vi "IQ Impairments impl.vi"(0 "session in":T1 {"rx baseband session"."3630 session"."Address Space" items=["VXI/VME A16"=1, "VXI/VME A24"=2, "VXI/VME A32"=3, "VXI/VME A64"=4, "PXI Memory Allocations"=9, "PXI Configuration"=10, "PXI BAR0"=11, "PXI BAR1"=12, "PXI BAR2"=13, "PXI BAR3"=14, "PXI BAR4"=15, "PXI BAR5"=16]; "tx baseband session"."3610 session"."Address Space" items=["VXI/VME A16"=1, "VXI/VME A24"=2, "VXI/VME A32"=3, "VXI/VME A64"=4, "PXI Memory Allocations"=9, "PXI Configuration"=10, "PXI BAR0"=11, "PXI BAR1"=12, "PXI BAR2"=13, "PXI BAR3"=14, "PXI BAR4"=15, "PXI BAR5"=16]}, 1 "direction":T12, 7 "device configuration":T15 {"Tx hardware configuration"."frequency (Hz)" format="%#_6p"; "Rx hardware configuration"."frequency (Hz)" format="%#_6p"}, 9 "IQ Impairments":T18[](array[typedef]) {"Phase Offset (radians)" format="%#_6f"; "Gain Imbalance (linear)" format="%#_6f"}, 11 "error in (no error)":errorcluster) -> (3 "scope":string[](array[string]), 4 "session out":T1 {"rx baseband session"."3630 session"."Address Space" items=["VXI/VME A16"=1, "VXI/VME A24"=2, "VXI/VME A32"=3, "VXI/VME A64"=4, "PXI Memory Allocations"=9, "PXI Configuration"=10, "PXI BAR0"=11, "PXI BAR1"=12, "PXI BAR2"=13, "PXI BAR3"=14, "PXI BAR4"=15, "PXI BAR5"=16]; "tx baseband session"."3610 session"."Address Space" items=["VXI/VME A16"=1, "VXI/VME A24"=2, "VXI/VME A32"=3, "VXI/VME A64"=4, "PXI Memory Allocations"=9, "PXI Configuration"=10, "PXI BAR0"=11, "PXI BAR1"=12, "PXI BAR2"=13, "PXI BAR3"=14, "PXI BAR4"=15, "PXI BAR5"=16]}, 6 "configuration gain":dbl[](array[numeric]), 8 "Index":i32[](array[numeric]), 14 "gain (db)":dbl[](array[numeric]), 15 "error out":errorcluster)   [LabVIEW 2019]
uses:
  <instrlib>/niMmWave/ni3620/Config/v1/Host/Public/Corrections/Typedefs/Opera IQ Impairment Data.ctl
  TypeDefs/Direction.ctl
  TypeDefs/Front End Configuration.ctl
  TypeDefs/Channel Configuration.ctl
  <instrlib>/niMmWave/ni3620/Config/v1/Host/Public/Typedefs/mmWave Port.ctl
  TypeDefs/Session.ctl
  <instrlib>/niMmWave/ni3620/Config/v1/Host/Public/High-Level/niMmWave Session.ctl
  <instrlib>/_niInstr/Register Bus/v0/Host/Public/Register Bus Session.ctl
  <instrlib>/_niInstr/Register Bus/v0/Host/Private/Session Data.ctl
  <instrlib>/niMmWave/ni3620/Config/v1/Host/Public/Typedefs/Board Information.ctl
  <instrlib>/niMmWave/ni3620/Config/v1/Host/Public/Typedefs/Hardware Revision.ctl
  <instrlib>/niMmWave/ni3620/Config/v1/Host/Public/Typedefs/Gain Mapping.ctl
  <instrlib>/niMmWave/ni3620/Config/v1/Host/Public/Typedefs/Correction Data.ctl
  <instrlib>/niMmWave/ni3620/Config/v1/Host/Public/Typedefs/Opera Characterization.ctl
  <instrlib>/niMmWave/ni3620/Config/v1/Host/Public/Corrections/Typedefs/Opera Characterization Main Header.ctl
  <instrlib>/niMmWave/ni3620/Config/v1/Host/Public/Corrections/Typedefs/Opera IF Board Information.ctl
  <instrlib>/niMmWave/ni3620/Config/v1/Host/Public/Corrections/Typedefs/Opera Characterization Instance Header.ctl
  <instrlib>/niMmWave/ni3620/Config/v1/Host/Public/Corrections/Typedefs/Opera Characterization Device Data Header.ctl
  <instrlib>/niMmWave/ni3620/Config/v1/Host/Public/Corrections/Typedefs/Opera LO Characterization Data Header.ctl
  <instrlib>/niMmWave/ni3620/Config/v1/Host/Public/Corrections/Typedefs/Opera IF Board Characterization Data Header.ctl
  <instrlib>/niMmWave/ni3620/Config/v1/Host/Public/Corrections/Typedefs/Opera Characterization Device Data.ctl
  <instrlib>/niMmWave/ni3620/Config/v1/Host/Public/Corrections/Typedefs/Opera LO2 Board Characterization Data.ctl
  <instrlib>/niMmWave/ni3620/Config/v1/Host/Public/Corrections/Typedefs/Opera LO Characterization Data.ctl
  <instrlib>/niMmWave/ni3620/Config/v1/Host/Public/Corrections/Typedefs/Opera IF Board Characterization Data.ctl
  <instrlib>/niMmWave/ni3620/Config/v1/Host/Public/Typedefs/mmWave Adapter Session Data.ctl
  <instrlib>/niMmWave/ni3620/Config/v1/Host/Public/Typedefs/mmWave Adapter Data.ctl
  <instrlib>/niMmWave/ni3620/Config/v1/Host/Public/Typedefs/mmWave Adapter 2.ctl
  <instrlib>/niMmWave/ni3620/Config/v1/Shared/Typedefs/Subsystem ID.ctl
  <instrlib>/niMmWave/ni3620/Config/v1/Host/Public/Typedefs/mmWave Adapter Channel Information.ctl
  <instrlib>/niMmWave/ni3620/Config/v1/Host/Public/Typedefs/Temperature Coefficients.ctl
  <instrlib>/niMmWave/ni3620/Config/v1/Host/Public/Typedefs/mmWave Characterization.ctl
  <instrlib>/niMmWave/ni3620/Config/v1/Host/Public/Corrections/Typedefs/mmWave Characterization Main Header.ctl
  <instrlib>/niMmWave/ni3620/Config/v1/Host/Public/Corrections/Typedefs/mmWave Characterization Instance Header.ctl
  <instrlib>/niMmWave/ni3620/Config/v1/Host/Public/Typedefs/Session Cache.ctl
  <instrlib>/niMmWave/ni3620/Config/v1/Host/Public/Typedefs/LO2 settings cache.ctl
  <instrlib>/niMmWave/ni3620/Config/v1/Host/Public/Typedefs/LO2 source.ctl
  <instrlib>/niMmWave/ni3620/Config/v1/Host/Public/Typedefs/Desired and Coerced.ctl
  <instrlib>/niMmWave/ni3620/Config/v1/Host/Public/Typedefs/Export cache.ctl
  <instrlib>/niMmWave/ni3620/Config/v1/Host/Public/Typedefs/Path cache.ctl
  <instrlib>/niMmWave/ni3620/Config/v1/Host/Public/Typedefs/Daughterboard Type.ctl
  <instrlib>/niMmWave/ni3620/Config/v1/Host/Public/Typedefs/LO1 settings cache.ctl
  <instrlib>/niMmWave/ni3620/Config/v1/Host/Public/Typedefs/LO1 Source.ctl
  <instrlib>/niMmWave/ni3620/Config/v1/Host/Public/Typedefs/mmWave export cache.ctl
  <instrlib>/niMmWave/ni3620/Config/v1/Host/Private/Board/LO2/LO2 Board Configuration Cache.ctl
  <instrlib>/niMmWave/ni3620/Config/v1/Host/Public/Typedefs/reference clock routing settings.ctl
  <instrlib>/niMmWave/ni3620/Config/v1/Host/Public/Typedefs/LO2 routing settings.ctl
  <instrlib>/niMmWave/ni3620/Config/v1/Host/Private/Board/LO1/LO1 Board Configuration Cache.ctl
  <instrlib>/niMmWave/ni3620/Config/v1/Host/Public/Typedefs/LO1 source settings.ctl
  <instrlib>/niMmWave/ni3620/Config/v1/Host/Public/Typedefs/LO1 export settings.ctl
  <instrlib>/niMmWave/ni3620/Config/v1/Host/Public/Typedefs/LO1 mmWave settings.ctl
  TypeDefs/Tx Baseband Session.ctl
  <instrlib>/niMmWave/ni3610 and ni3630/controls/public/Main Settings.ctl
  <vilib>/Instr/_visa.llb/VISA Register Access Address Space.ctl
  <instrlib>/niMmWave/ni3610 and ni3630/controls/public/Register Adresses.ctl
  <instrlib>/niMmWave/ni3610 and ni3630/controls/public/Base Card Type.ctl
  <instrlib>/niMmWave/ni3610 and ni3630/controls/private/IQ Card Revision.ctl
  <instrlib>/niMmWave/ni3610 and ni3630/controls/public/Board Capability.ctl
  TypeDefs/Blank FPGA Reference.ctl
  TypeDefs/Rx Baseband Session.ctl
  TypeDefs/Hardware Configuration.ctl
  TypeDefs/Gain Ranging.ctl
  TypeDefs/PXI Trigger Bus Info.ctl
  TypeDefs/Shared FPGA Reference.ctl
  <vilib>/Utility/error.llb/Error Cluster From Error Code.vi
  <vilib>/rvi/errors/niLvFpgaAdjustHostInterfaceError.vi
  <vilib>/rvi/interface/nirviReadWriteControl/nirviReadWriteControl.xnode
  NiFpgaLv.dll
  <vilib>/rvi/interface/Simulation/niFpgaSimulationCallBeginRW.vi
  <instrlib>/niMmWave/ni3620/Config/v1/Host/niMmWave Config v1 Host.lvlib
  <instrlib>/niMmWave/ni3620/Config/v1/Shared/niMmWave Config v1 Shared.lvlib
  <instrlib>/_niInstr/Register Bus/v0/Host/niInstr Register Bus v0 Host.lvlib
  <instrlib>/niMmWave/ni3610 and ni3630/ni3610_and_ni3630_Driver_Lib.lvlib
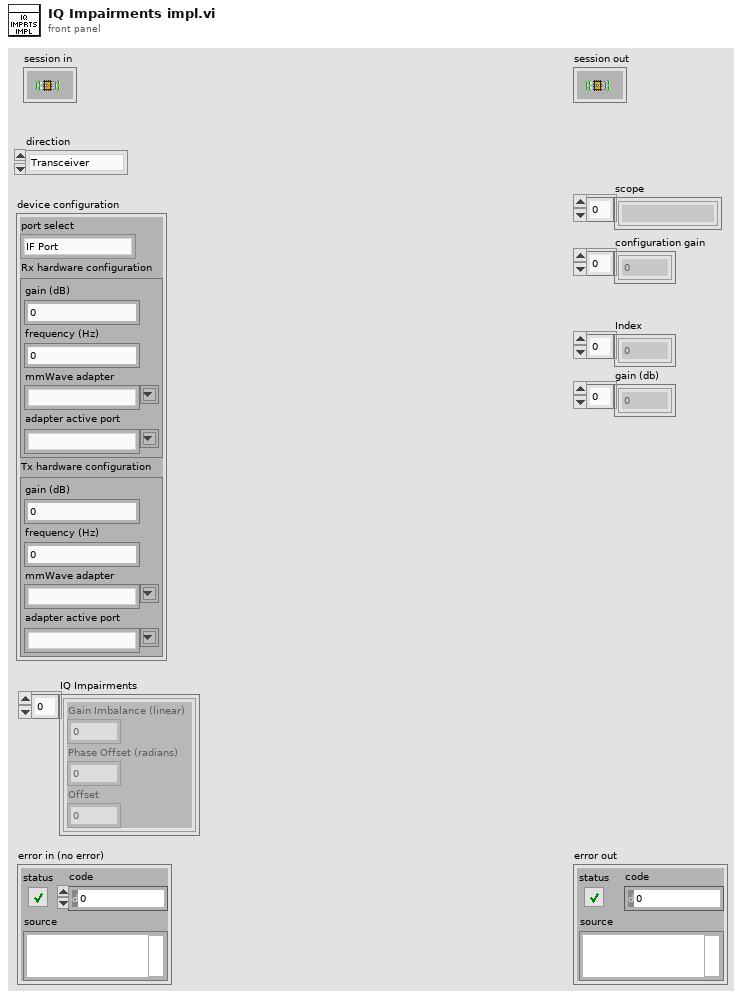
[diagram p1: front panel]
types:
  T1 = typedef "Session.ctl" = cluster{"3620 session":refnum<queue>, "tx baseband session":T2, "rx baseband session":T10, "tx gain (dB)":dbl, "rx gain (dB)":dbl, "hardware configuration":T11, "gain ranging":T13[], "pxi trigger bus information":T14}
  T2 = typedef "Tx Baseband Session.ctl" = cluster{"3610 session":T3, "7902 reference":T9}
  T3 = typedef "ni3610_and_ni3630_Driver_Lib.lvlib/Main Settings.ctl" = cluster{"VISA resource name":refnum<visa-resource-name>, "Address Space":T4, "window_offset":u32, "register_addresses":T5, "required_MM_fpga_version":cluster{"signature":u32, "hardware":u32, "current revision":u32, "oldest revision":u32}, "CPLD Oldest Compat Version ":cluster{"hardware":u32, "CPLD firmware":u32}, "MM_FPGA_image_location":string, "is_init":bool, "card_type":T6, "DacLmkConfigFileName":string, "AdcLmkConfigFileName":string, "AdcConfigFileName":string, "DacConfigFileName_RevA":string, "DacConfigFileName_RevB":string, "Mulde hardware revision":u8, "bypass DAC PLL\n":bool, "IQ Card Revision":T7, "board capability":T8}
  T4 = typedef "VISA Register Access Address Space.ctl" = u16
  T5 = typedef "ni3610_and_ni3630_Driver_Lib.lvlib/Register Adresses.ctl" = cluster{"MM based Registers":cluster{"Revision":u32, "OldestCompatRev":u32, "signature":u32, "scratch":u32, "LedControl":u32, "BoardHwRev":u32, "BoardControl":u32, "ThermalStatus":u32, "BasebandStatus":u32, "BasebandControl":u32, "BasebandAuxSetup":u32, "BasebandAuxStatus":u32, "LmkSyncOutSetup":u32, " AdcSyncOutSetup":u32, " InjSyncOutSetup":u32, " PxiTrig0OutSetup":u32, " PxiTrig1OutSetup":u32, " PxiTrig2OutSetup":u32, " PxiTrig3OutSetup":u32, " PxiTrig4OutSetup":u32, " PxiTrig5OutSetup":u32, " PxiTrig6OutSetup":u32, " PxiTrig7OutSetup":u32}, "CPLD based Registers":cluster{"SlaveSignature":u32, "SlaveRevision":u32, "SlaveOldestCompatRev":u32, "SlaveScratch":u32, "SlaveSetup":u32, "SlaveStatus":u32, "IDacReg_offset":u32, "LMKRegGrp0_offset":u32, "QDacReg_offset":u32, "BrdTempSensorVal":u32, "TempSensorPowerDown":u32, "GPIOReg_offset":u32, "IAdcReg_offset":u32, "QAdcReg_offset":u32, "LMKRegGrp1_offset":u32, "QadcTempSensorVal":u32, "IadcTempSensorVal":u32, "RevisionReg":u32, "VcxoReg":u32, "CpldStatusReg":u32, "PowerReg":u32, "VBiasEnReg":u32, "ExtRefOeReg":u32, "QdacCtrlReg":u32, "QdacStatusReg":u32, "IdacCtrlReg":u32, "IdacStatusReg":u32, "QdacJtagIn":u32, "QdacJtagOut":u32, "IdacJtagIn":u32, "IdacJtagOut":u32, "IqDcSetupReg":u32, "QadcStatusReg":u32, "IadcStatusReg":u32, "BrdSetupReg":u32, "IqDcRevisionReg":u32, "PllStatusReg":u32, "EndpointScratchReg":u32, "AdcSyncCfgReg":u32, "IqCardOpampReg":u32}, "CPLD Register Offset":u32, "MM  Register Offset":u32, " PxiTrig0OutSetup":u32}
  T6 = typedef "ni3610_and_ni3630_Driver_Lib.lvlib/Base Card Type.ctl" = enum16{"unspecified", "ADC", "DAC"}
  T7 = typedef "ni3610_and_ni3630_Driver_Lib.lvlib/IQ Card Revision.ctl" = enum16{"RevA", "RevB", "RevC", "RevD"}
  T8 = typedef "ni3610_and_ni3630_Driver_Lib.lvlib/Board Capability.ctl" = cluster{"baseband sync":enum16{"no baseband sync", "baseband sync"}}
  T9 = typedef "Blank FPGA Reference.ctl" = refnum<k20>
  T10 = typedef "Rx Baseband Session.ctl" = cluster{"3630 session":T3, "7902 reference":T9}
  T11 = typedef "Hardware Configuration.ctl" = cluster{"direction":T12, "baseband only":bool}
  T12 = typedef "Direction.ctl" = enum16{"Transceiver", "Receiver", "Transmitter"}
  T13 = typedef "Gain Ranging.ctl" = cluster{"gain ranging active scope":string, "gain ranging stream session":refnum<k20>}
  T14 = typedef "PXI Trigger Bus Info.ctl" = cluster{"chassis resource name":refnum<visa-resource-name>, "7902R (TX)":i16, "3610 (TX)":i16, "3620 (IF)":i16, "3630 (RX)":i16, "7902R (RX)":i16}
  T15 = typedef "Front End Configuration.ctl" = cluster{"port select":enum16{"IF Port", "Loopback", "Sync Port"}, "Rx hardware configuration":T16, "Tx hardware configuration":T16}
  T16 = typedef "Channel Configuration.ctl" = cluster{"gain (dB)":dbl, "frequency (Hz)":dbl, "mmWave adapter":string, "adapter active port":T17}
  T17 = typedef "niMmWave Config v1 Host.lvlib/mmWave Port.ctl" = string
  T18 = typedef "niMmWave Config v1 Host.lvlib/Opera IQ Impairment Data.ctl" = cluster{"Gain Imbalance (linear)":dbl, "Phase Offset (radians)":dbl, "Offset ":cdb}
  T19 = typedef "Shared FPGA Reference.ctl" = refnum<k20>
  T20 = cluster{"sample delay":cluster{"I delay":fxp<+,13,13>, "Q delay":fxp<+,13,13>}, "fractional delay":cluster{"enable":bool, "coef write":bool, "coef data":fxp<+/-,18,1>}, "impairments":cluster{"inline gain I":fxp<+/-,18,1>, "inline gain Q":fxp<+/-,18,1>, "cross gain I":fxp<+/-,18,1>, "cross gain Q":fxp<+/-,18,1>, "pre-gain offset I":fxp<+/-,18,1>, "pre-gain offset Q":fxp<+/-,18,1>, "post-gain offset I":fxp<+/-,18,1>, "post-gain offset Q":fxp<+/-,18,1>}, "iq inversion":cluster{"invert I":bool, "invert Q":bool}}
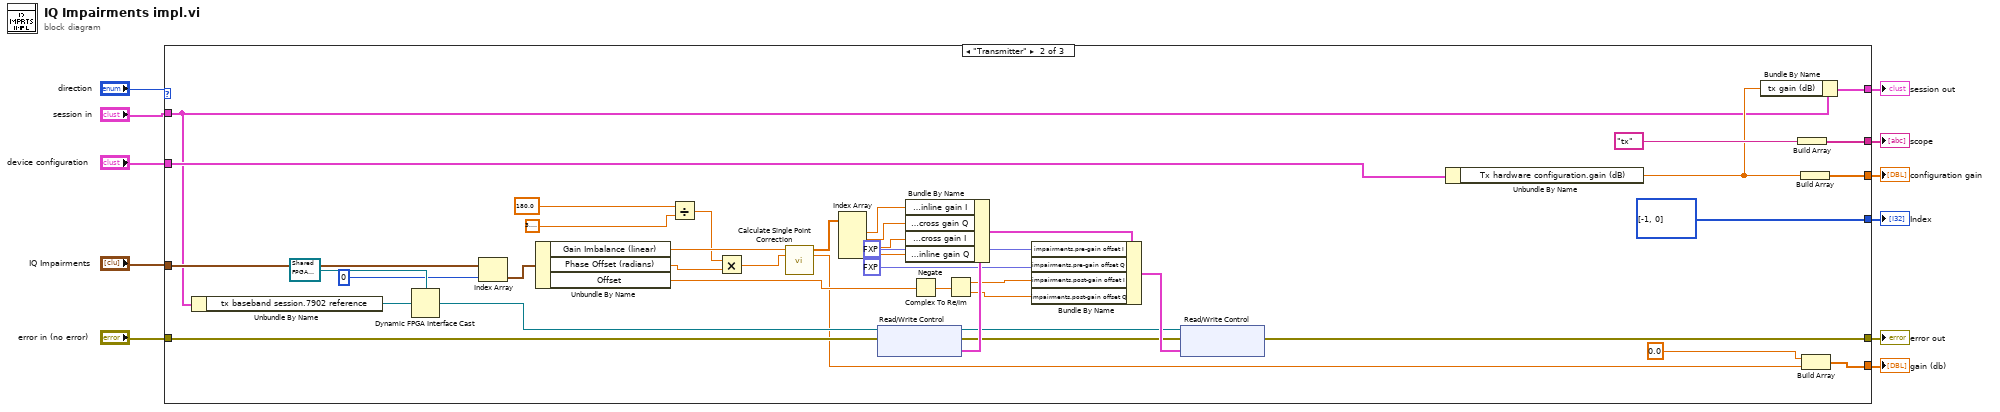
[diagram p0: block diagram]
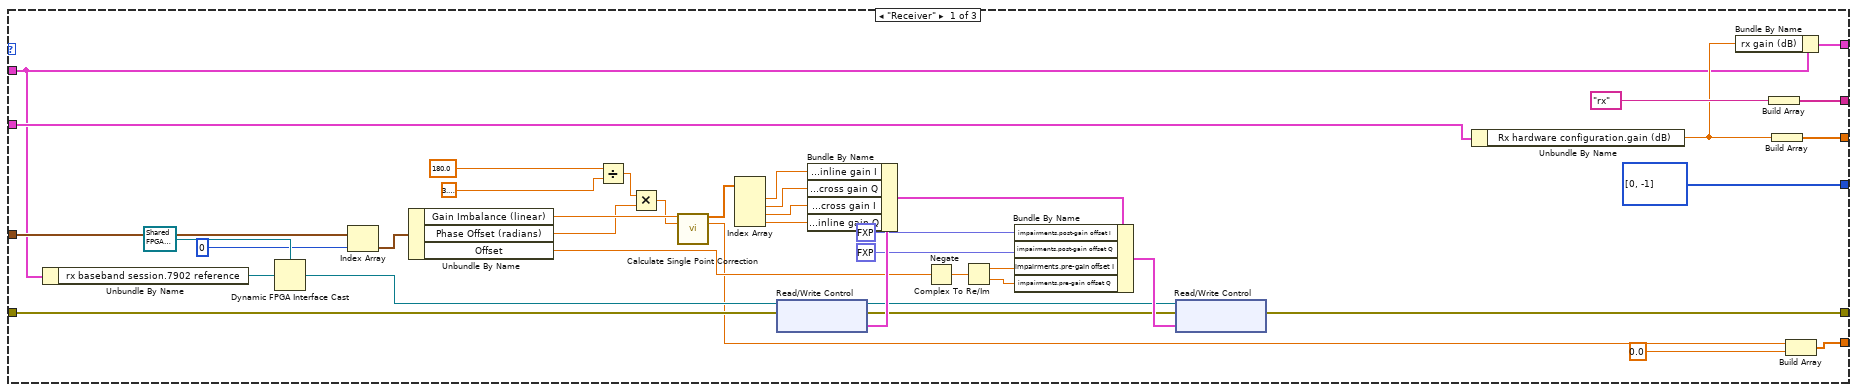
[diagram p2: hidden frame]
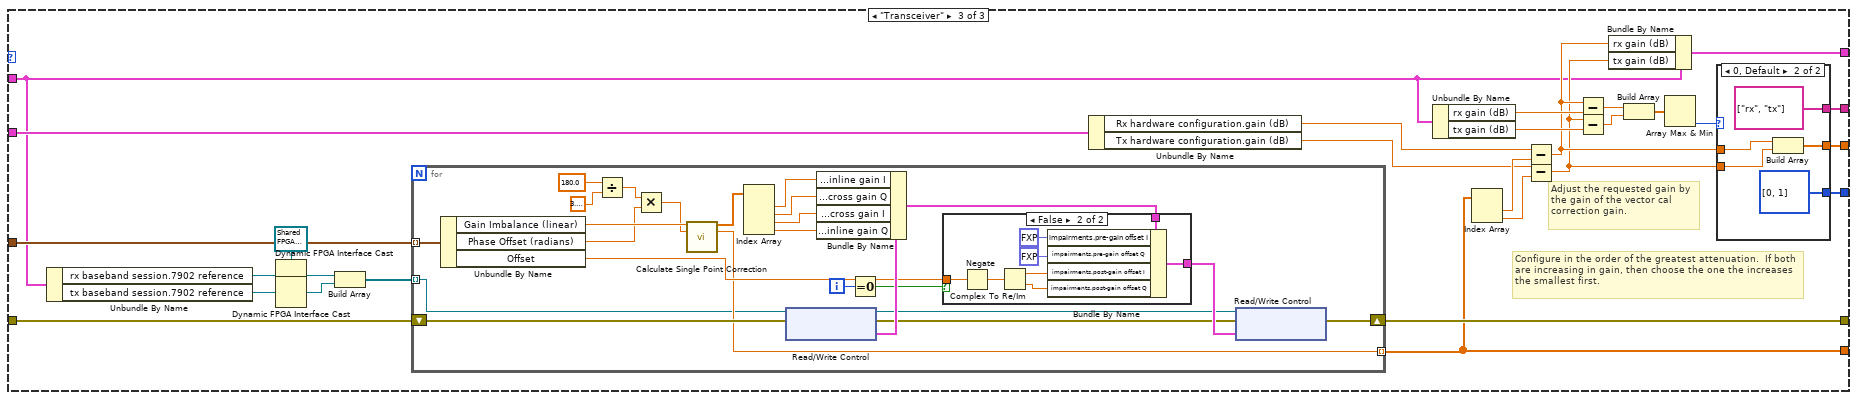
[diagram p3: hidden frame]
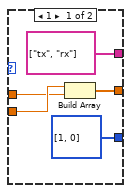
[diagram p4: hidden frame]
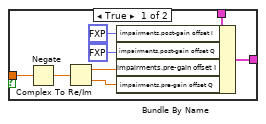
[diagram p5: hidden frame]
diagram:
  n1 = case shown="\"Transmitter\"" "direction" {
    tunnel: [w50 w91 w121] -> w5
    tunnel: [w52 w93 w120] -> w4
    tunnel: "device configuration" -> [w49 w90 w95]
    tunnel: "session in" -> [w12 w53 w94]
    tunnel: [i32[] [0, -1] i32[] [-1, 0] w114] -> w3
    tunnel: [w47 w88 w113] -> w6
    tunnel: [w26 w64 w109] -> w2
    tunnel: "error in (no error)" -> [w27 w65 w110]
    tunnel: "IQ Impairments" -> [w42 w66 w97]
    tunnel: [w23 w61 w96] -> w1
    frame "Receiver" {
      n2 = Unbundle By Name(w12) -> ("rx baseband session.7902 reference"=w44:T9)
      n3 = Dynamic FPGA Interface Cast(Session In=T19 refnum ("fpga reference"), Type=w44) -> (Session Out=w43:T19)
      n4 = Index Array(array=w42, index=0) -> (element=w40:T18)
      n5 = Unbundle By Name(w40) -> ("Gain Imbalance (linear)"=w34:dbl, "Phase Offset (radians)"=w14:dbl, "Offset"=w31:cdb)
      n6 = Divide(x=180.0, y=3.141592653589793) -> (x/y=w15:dbl)
      n7 = Multiply(x=w15, y=w14) -> (x*y=w13:dbl)
      n8 = call "Calculate Single Point Correction.vi"("gain imbalance"=w34, "phase skew"=w13) -> ("matrix coefficients"=w35:dbl[], "gain (dB)"=w25:dbl)  [unwired: 11 in, 1 out]
      n9 = Index Array(array=w35) -> (element #1=w39:dbl, element #2=w38:dbl, element #3=w37:dbl, element #4=w36:dbl)  [unwired: 4 in]
      n10 = xnode "Read/Write Control"("FPGA VI Reference In"=w43, "error in"=w27) -> ("FPGA VI Reference Out"=w28:T19, "error out"=w29:errorcluster, "cal.correction"=w33:T20)
      n11 = Bundle By Name(cluster=w33, "impairments.inline gain I"=w39, "impairments.cross gain Q"=w38, "impairments.cross gain I"=w37, "impairments.inline gain Q"=w36) -> (w32:T20)
      n12 = Negate(x=w31) -> (-x=w22:cdb)
      n13 = Complex To Re/Im(x + iy=w22) -> (x=w21:dbl, y=w20:dbl)
      n14 = Bundle By Name(cluster=w32, "impairments.post-gain offset I"=fxp<+/-,18,1> 0.0, "impairments.post-gain offset Q"=fxp<+/-,18,1> 0.0, "impairments.pre-gain offset I"=w21, "impairments.pre-gain offset Q"=w20) -> (w30:T20)
      n15 = xnode "Read/Write Control"("FPGA VI Reference In"=w28, "error in"=w29, "cal.correction"=w30) -> ("error out"=w26:errorcluster)  [unwired: 1 out]
      n16 = Unbundle By Name(w49) -> ("Rx hardware configuration.gain (dB)"=w46:dbl)
      n17 = Bundle By Name(cluster=w12, "rx gain (dB)"=w46) -> (w47:T1)
      n18 = Build Array("rx" ("scope")) -> (w50:string[])
      n19 = Build Array(w46) -> (w52:dbl[])
      n20 = Build Array(w25, 0.0 ("element")) -> (w23:dbl[])
    }
    frame "Transmitter" {
      n21 = Unbundle By Name(w53) -> ("tx baseband session.7902 reference"=w85:T9)
      n22 = Dynamic FPGA Interface Cast(Session In=T19 refnum ("fpga reference"), Type=w85) -> (Session Out=w84:T19)
      n23 = Index Array(array=w66, index=0) -> (element=w82:T18)
      n24 = Unbundle By Name(w82) -> ("Gain Imbalance (linear)"=w76:dbl, "Phase Offset (radians)"=w55:dbl, "Offset"=w73:cdb)
      n25 = Divide(x=180.0, y=3.141592653589793) -> (x/y=w56:dbl)
      n26 = Multiply(x=w56, y=w55) -> (x*y=w54:dbl)
      n27 = call "Calculate Single Point Correction.vi"("gain imbalance"=w76, "phase skew"=w54) -> ("matrix coefficients"=w77:dbl[], "gain (dB)"=w63:dbl)  [unwired: 11 in, 1 out]
      n28 = Index Array(array=w77) -> (element #1=w81:dbl, element #2=w80:dbl, element #3=w79:dbl, element #4=w78:dbl)  [unwired: 4 in]
      n29 = xnode "Read/Write Control"("FPGA VI Reference In"=w84, "error in"=w65) -> ("FPGA VI Reference Out"=w70:T19, "error out"=w71:errorcluster, "cal.correction"=w75:T20)
      n30 = Bundle By Name(cluster=w75, "impairments.inline gain I"=w81, "impairments.cross gain Q"=w80, "impairments.cross gain I"=w79, "impairments.inline gain Q"=w78) -> (w74:T20)
      n31 = Negate(x=w73) -> (-x=w69:cdb)
      n32 = Complex To Re/Im(x + iy=w69) -> (x=w68:dbl, y=w67:dbl)
      n33 = Bundle By Name(cluster=w74, "impairments.pre-gain offset I"=fxp<+/-,18,1> 0.0, "impairments.pre-gain offset Q"=fxp<+/-,18,1> 0.0, "impairments.post-gain offset I"=w68, "impairments.post-gain offset Q"=w67) -> (w72:T20)
      n34 = xnode "Read/Write Control"("FPGA VI Reference In"=w70, "error in"=w71, "cal.correction"=w72) -> ("error out"=w64:errorcluster)  [unwired: 1 out]
      n35 = Unbundle By Name(w90) -> ("Tx hardware configuration.gain (dB)"=w87:dbl)
      n36 = Bundle By Name(cluster=w53, "tx gain (dB)"=w87) -> (w88:T1)
      n37 = Build Array("tx" ("scope")) -> (w91:string[])
      n38 = Build Array(w87) -> (w93:dbl[])
      n39 = Build Array(0.0 ("element"), w63) -> (w61:dbl[])
    }
    frame "Transceiver" {
      w104 = T19 refnum ("fpga reference")
      # "Configure in the order of the greatest attenuation.  If both are increasing in gain, then choose the one the increases the smallest first."
      # "Adjust the requested gain by the gain of the vector cal correction gain."
      n40 = Unbundle By Name(w94) -> ("rx baseband session.7902 reference"=w111:T9, "tx baseband session.7902 reference"=w108:T9)
      n41 = Dynamic FPGA Interface Cast(Session In=w104, Type=w111) -> (Session Out=w107:T19)
      n42 = Dynamic FPGA Interface Cast(Session In=w104, Type=w108) -> (Session Out=w106:T19)
      n43 = Build Array(w107, w106) -> (w105:T19[])
      n44 = for {
        shift-right: [w139] -> w109
        shift-left: w110 -> [w142]
        tunnel: w105 -> [w137] mode=indexing
        tunnel: [w140] -> w96 mode=indexing
        tunnel: w97 -> [w138] mode=indexing
        i -> [w141]
        n45 = Unbundle By Name(w138) -> ("Gain Imbalance (linear)"=w150:dbl, "Phase Offset (radians)"=w134:dbl, "Offset"=w147:cdb)
        n46 = Divide(x=180.0, y=3.141592653589793) -> (x/y=w133:dbl)
        n47 = Multiply(x=w133, y=w134) -> (x*y=w132:dbl)
        n48 = call "Calculate Single Point Correction.vi"("gain imbalance"=w150, "phase skew"=w132) -> ("matrix coefficients"=w151:dbl[], "gain (dB)"=w140:dbl)  [unwired: 11 in, 1 out]
        n49 = Index Array(array=w151) -> (element #1=w155:dbl, element #2=w154:dbl, element #3=w153:dbl, element #4=w152:dbl)  [unwired: 4 in]
        n50 = xnode "Read/Write Control"("FPGA VI Reference In"=w137, "error in"=w142) -> ("FPGA VI Reference Out"=w144:T19, "error out"=w145:errorcluster, "cal.correction"=w149:T20)
        n51 = Bundle By Name(cluster=w149, "impairments.inline gain I"=w155, "impairments.cross gain Q"=w154, "impairments.cross gain I"=w153, "impairments.inline gain Q"=w152) -> (w148:T20)
        n52 = Equal To 0?(x=w141) -> (x = 0?=w143:bool)
        n53 = case shown="False" w143 {
          tunnel: w148 -> [w162 w170]
          tunnel: w147 -> [w159 w168]
          tunnel: [w158 w167] -> w146
          frame True {
            n54 = Negate(x=w159) -> (-x=w163:cdb)
            n55 = Complex To Re/Im(x + iy=w163) -> (x=w161:dbl, y=w160:dbl)
            n56 = Bundle By Name(cluster=w162, "impairments.post-gain offset I"=fxp<+/-,18,1> 0.0, "impairments.post-gain offset Q"=fxp<+/-,18,1> 0.0, "impairments.pre-gain offset I"=w161, "impairments.pre-gain offset Q"=w160) -> (w158:T20)
          }
          frame False {
            n57 = Negate(x=w168) -> (-x=w171:cdb)
            n58 = Complex To Re/Im(x + iy=w171) -> (x=w169:dbl, y=w166:dbl)
            n59 = Bundle By Name(cluster=w170, "impairments.pre-gain offset I"=fxp<+/-,18,1> 0.0, "impairments.pre-gain offset Q"=fxp<+/-,18,1> 0.0, "impairments.post-gain offset I"=w169, "impairments.post-gain offset Q"=w166) -> (w167:T20)
          }
        }
        n60 = xnode "Read/Write Control"("FPGA VI Reference In"=w144, "error in"=w145, "cal.correction"=w146) -> ("error out"=w139:errorcluster)  [unwired: 1 out]
      }
      n61 = Unbundle By Name(w95) -> ("Rx hardware configuration.gain (dB)"=w101:dbl, "Tx hardware configuration.gain (dB)"=w99:dbl)
      n62 = Unbundle By Name(w94) -> ("rx gain (dB)"=w119:dbl, "tx gain (dB)"=w112:dbl)
      n63 = Index Array(array=w96) -> (element #1=w103:dbl, element #2=w102:dbl)  [unwired: 2 in]
      n64 = Subtract(x=w101, y=w103) -> (x-y=w100:dbl)
      n65 = Subtract(x=w99, y=w102) -> (x-y=w98:dbl)
      n66 = Subtract(x=w100, y=w119) -> (x-y=w118:dbl)
      n67 = Subtract(x=w98, y=w112) -> (x-y=w117:dbl)
      n68 = Bundle By Name(cluster=w94, "rx gain (dB)"=w100, "tx gain (dB)"=w98) -> (w113:T1)
      n69 = Build Array(w118, w117) -> (w116:dbl[])
      n70 = Array Max & Min(array=w116) -> (min index (indices)=w115:i32)  [unwired: 3 out]
      n71 = case shown="0, Default" w115 {
        tunnel: w100 -> [w123 w129]
        tunnel: w98 -> [w124 w128]
        tunnel: [string[] ["tx", "rx"] string[] ["rx", "tx"]] -> w121
        tunnel: [w125 w130] -> w120
        tunnel: [i32[] [1, 0] i32[] [0, 1]] -> w114
        frame 1 {
          n72 = Build Array(w124, w123) -> (w125:dbl[])
        }
        frame 0, Default {
          n73 = Build Array(w129, w128) -> (w130:dbl[])
        }
      }
    }
  }
  "session out" <- w6
  "scope" <- w5
  "configuration gain" <- w4
  "Index" <- w3
  "error out" <- w2
  "gain (db)" <- w1
